vi "Clear Filters.vi"(8 "error in (no error)":errorcluster, 11 "Error Manager in":refnum<class "Error Manager.lvclass">) -> (0 "error out":errorcluster, 2 "Filters to clear":set{i32}(c389), 3 "Error Manager out":refnum<class "Error Manager.lvclass">)   [LabVIEW 2026, in "TALOS.lvlib" / "Error Manager.lvlib" / "Error Manager.lvclass"]
uses:
  Error Manager.lvclass
  C:/LabVIEW Code/TALOS/talos/Father of all uServices/Father of all uServices/Father of all uServices.lvclass
  Error Manager.lvclass/Error Manager.ctl
  Father of all uServices/Father of all uServices/Father of all uServices.lvclass/Father of all uServices.ctl
  Ancestor/Ancestor/Ancestor.lvclass/Ancestor.ctl
  Support VIs/Substitute Error.vi
  Support VIs/Generate Error.vi
  FGV/Error Memory/Get Error Description.vi
  Support VIs/Get PC name.vi
  Ancestor/Ancestor/Read ID.vi
  Support VIs/Get Class Name.vi
  <vilib>/Utility/error.llb/Clear Errors.vi
  FGV/Error Memory/Error Memory Core.vi
  <vilib>/AdvancedString/Delimited String to 1D String Array.vi
  <vilib>/AdvancedString/Delimited String to 1D String Array (string).vi
  Support VIs/Circus Root Path.vi
  FGV/Error Memory/Error Crt Lvl checker.vi
  FGV/Error Memory/Error Memory Core.vi/40c8088d-b597-4017-91af-faa98e00292e.vi
  FGV/Error Memory/Error Memory Core.vi/d4a3ab98-063c-4e44-b43d-fbdcfe6c2be2.vi
  Support VIs/Global Memory.vi
  <vilib>/Utility/LVClass/Get LV Class Name.vi
  Support VIs/Is in Packed Library.vi
  Support VIs/TALOS Root path.vi
  Support VIs/Read CSV worksheet.vi
  Support VIs/Global Constants.vi
  <vilib>/Utility/error.llb/General Error Handler.vi
  Support VIs/Error Log.vi
  Ancestor/Ancestor/Ancestor.lvclass
  <vilib>/Comparison/Equal/Equal Functor/Equal Functor.lvclass
  Father of all uServices/Father of all uServices/Father of all uServices.lvclass
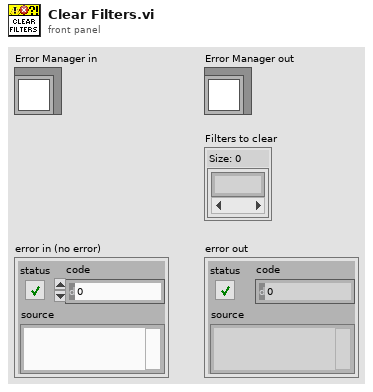
[diagram p1: front panel]
types:
  T1 = typedef "TALOS.lvlib/Error Manager.lvlib/Error Manager.lvclass/Error Info.ctl" = cluster{"error out":errorcluster, "Time Stamp":timestamp, "Machine Name":string, "GUID":string}
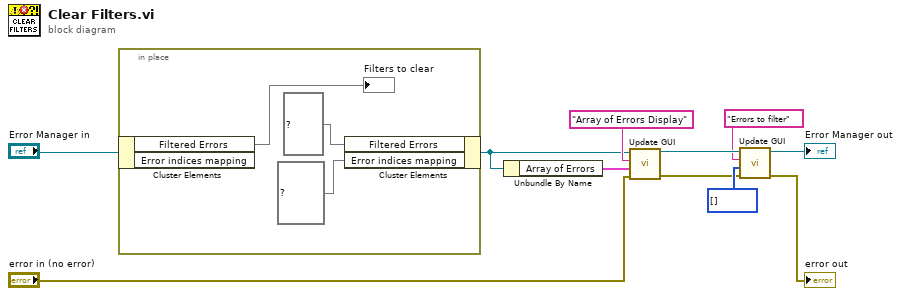
[diagram p0: block diagram]
diagram:
  n1 = in-place {
    n2 = in-place-cluster #1("Error Manager in") -> ("Filtered Errors"=→"Filters to clear":set{i32})  [unwired: 1 out]
    n3 = in-place-cluster #1("Filtered Errors"=set{i32} {}, "Error indices mapping"=map{i32, i32} {}) -> (w1:refnum<class "Error Manager.lvclass">)
  }
  n4 = Unbundle By Name(w1) -> ("Array of Errors"=w5:T1[])
  n5 = call "Update GUI.vi"("error in (no error)"="error in (no error)", "Data"=w5, "GUI Item Name"="Array of Errors Display" ("FP Item Name"), "uService Template in"=w1) -> ("error out"=w9:errorcluster, "uService Template out"=w7:refnum<class "Error Manager.lvclass">)  [unwired: 6 in]
  n6 = call "Update GUI.vi"("error in (no error)"=w9, "Data"=i32[] [], "GUI Item Name"="Errors to filter" ("FP Item Name"), "uService Template in"=w7) -> ("error out"=→"error out":errorcluster, "uService Template out"=→"Error Manager out":refnum<class "Error Manager.lvclass">)  [unwired: 6 in]
